vi "Remote VI Run.vi"(10 "VI Path":path) -> (3 "VI Reference":refnum<vi>)   [LabVIEW 2017]
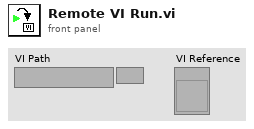
[diagram p1: front panel]
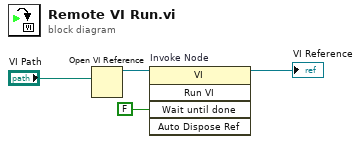
[diagram p0: block diagram]
diagram:
  n1 = Open VI Reference(vi path="VI Path") -> (vi reference=w2:refnum<vi>)  [unwired: 5 in, 1 out]
  n2 = invoke on="Invoke Node" class="VI" method="Run VI"(reference=w2, "Wait until done"=FALSE ("Wait Until Done")) -> (reference out=→"VI Reference":refnum<vi>)  [unwired: 3 in, 4 out]
